vi "Send Receive LaunchPad.vi"(0 "VISA resource":refnum<visa-resource-name>, 5 "write buffer":string, 7 "Bytes To Read (0)":u8, 9 "Max Retries  (10)":i32=10, 11 "error in":errorcluster, 12 "Time Out (100 ms)":i32=100) -> (4 "VISA resource 2":refnum<visa-resource-name>, 6 "Read Buffer":string, 15 "error out":errorcluster)   [LabVIEW 2012]
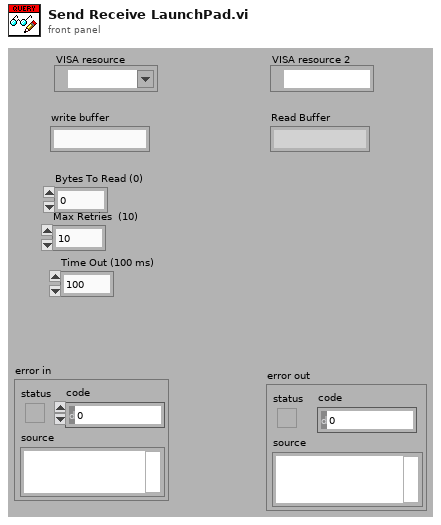
[diagram p1: front panel]
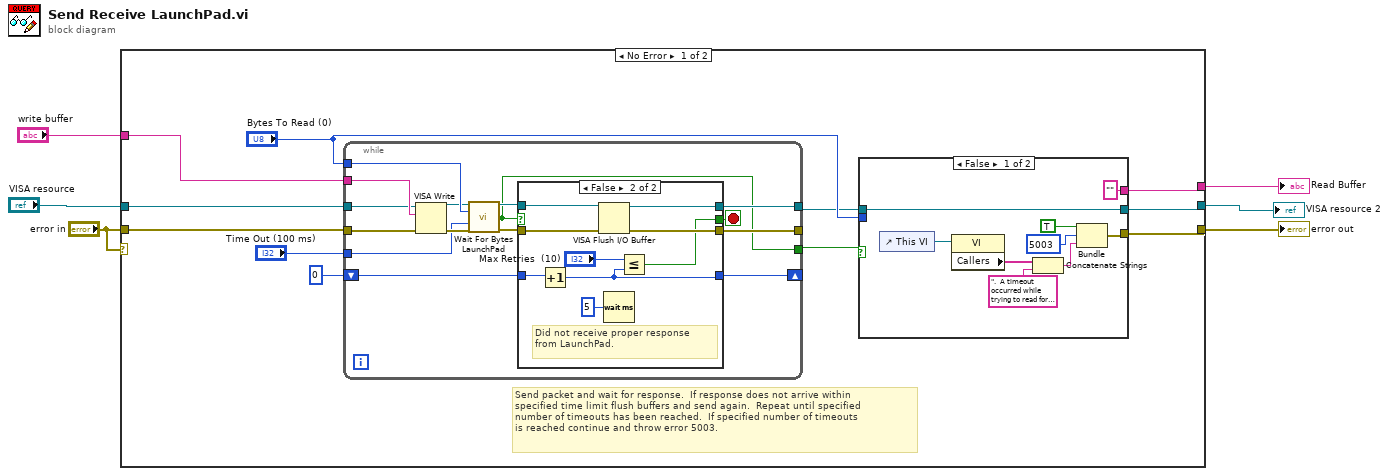
[diagram p0: block diagram]
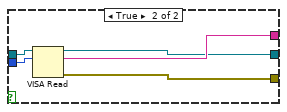
[diagram p3: hidden frame]
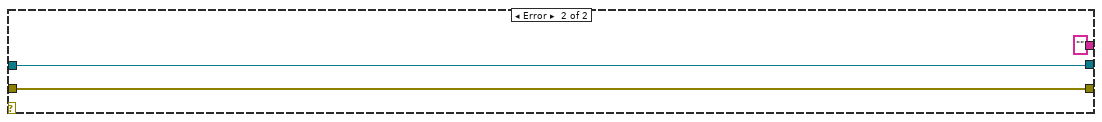
[diagram p4: hidden frame]
diagram:
  n1 = case shown="No Error" "error in" {
    tunnel: [w17 w62] -> w6
    tunnel: [w16 "" ("read buffer")] -> w5
    tunnel: "error in" -> [w12 w62]
    tunnel: "VISA resource" -> [w13 w60]
    tunnel: "write buffer" -> [w11 _]
    tunnel: [w10 w60] -> w1
    frame No Error {
      # "Send packet and wait for response.  If response does not arrive within \nspecified time limit flush buffers and send again.  Repeat until specified \nnumber of timeouts has been reached.  If specified number of timeouts\nis reached continue and throw error 5003."
      n2 = while {
        tunnel: w11 -> [w32]
        tunnel: [w26] -> w7
        tunnel: w12 -> [w31]
        tunnel: w13 -> [w30]
        tunnel: "Bytes To Read (0)" -> [w22]
        tunnel: "Time Out (100 ms)" -> [w23]
        tunnel: [w18] -> w9
        shift-right: [w28] -> _
        shift-left: 0 -> [w29]
        tunnel: [w25] -> _
        stop <- w27 stop-if-true
        n3 = VISA Write(VISA resource name=w30, write buffer=w32, error in (no error)=w31) -> (VISA resource name out=w21:refnum<visa-resource-name>, error out=w24:errorcluster)  [unwired: 1 out]
        n4 = call "Wait For Bytes LaunchPad.vi"("VISA resource"=w21, "Bytes To Read"=w22, "Time Out (100 ms)"=w23, "error in"=w24) -> ("VISA resource"=w20:refnum<visa-resource-name>, "Bytes Available?"=w18:bool, "error out"=w19:errorcluster)  [unwired: 9 in]
        n5 = case shown="False" w18 {
          selector: w18 -> [w35 _]
          tunnel: w29 -> [w36 w45]
          tunnel: [w36 w39] -> w28
          tunnel: [w35 w38] -> w27
          tunnel: w19 -> [w33 w43]
          tunnel: [w34 w42] -> w26
          tunnel: w20 -> [w34 w41]
          tunnel: [w33 w40] -> w25
          frame True {
          }
          frame False {
            # "Did not receive proper response\nfrom LaunchPad."
            n6 = Increment(x=w45) -> (x+1=w39:i32)
            n7 = VISA Flush I/O Buffer(VISA resource name=w41, error in (no error)=w43) -> (VISA resource name out=w42:refnum<visa-resource-name>, error out=w40:errorcluster)  [unwired: 1 in]
            n8 = Wait (ms)(milliseconds to wait=u32 5) -> ()  [unwired: 1 out]
            n9 = Less Or Equal?(x="Max Retries  (10)", y=w39) -> (x <= y?=w38:bool)
          }
        }
      }
      n10 = case shown="False" w9 {
        tunnel: [w49 w59] -> w17
        tunnel: ["" ("read buffer") w58] -> w16
        tunnel: w7 -> [w54 w57]
        tunnel: [w54 w56] -> w10
        tunnel: "Bytes To Read (0)" -> [_ w55]
        frame False {
          n11 = control-ref of="This VI"() -> (w50:refnum<vi>)
          n12 = property class="VI"(reference=w50) -> ("Callers"=w51:string[])  [unwired: 1 in, 2 out]
          n13 = Concatenate Strings(w51, ".  A timeout occurred while trying to read form the LaunchPad." ("string")) -> (w48:string)
          n14 = Bundle(TRUE, "code"=5003, w48) -> (w49:cluster{bool, "code":i32, string})  [unwired: 1 in]
        }
        frame True {
          n15 = VISA Read(VISA resource name=w57, byte count=w55) -> (VISA resource name out=w56:refnum<visa-resource-name>, read buffer=w58:string, error out=w59:errorcluster)  [unwired: 1 in, 1 out]
        }
      }
    }
    frame Error {
    }
  }
  "error out" <- w6
  "Read Buffer" <- w5
  "VISA resource 2" <- w1
